vi "P2022 TB INCAR GLOBALES.vi"() -> ()   [LabVIEW 2013]
uses:
  Controles/P2018 Com Control.ctl
  modbusEurotherm P116_485/P2018 Eurotherm Control.ctl
  modbusEurotherm P116_485/4xP116.ctl
  Controles/P2018 Bronkhorst Control.ctl
  serialBronkhorst/_s_TablaBronkhorst.ctl
  Controles/P2018 DisbalTB Control.ctl
  Controles/P2018 Arduino Control.ctl
panel:
  in  "TEMPERATURA":string
  in  "PESO":string
  in  "Cambia_F_f":bool
  out "ERRORES_BONKHORS_f":i32=5 caption="Elapsed Time (s)"
  in  "flowbus_MassFlow":T1={"Dispositivos"=[["3", "NO", "M0000013", "Air", "10", "ln/mn", "0", "0"], ["4", "NO", "M0000014", "Air", "10", "ln/mn", "0", "0"], ["5", "NO", "M0000015", "Air", "10", "ln/mn", "0", "0"], ["6", "NO", "M0000016", "Air", "10", "ln/mn", "0", "0"], ["7", "NO", "M0000017", "Air", "10", "ln/mn", "0", "0"], ["8", "NO", "M0000018", "Air", "10", "ln/mn", "0", "0"]], "NuevosSP"=[["0", "NO", "M0000013", "Air", "1", "ln/mn", "0", "0"], ["0", "NO", "M0000014", "Air", "1", "ln/mn", "0", "0"], ["0", "NO", "M0000015", "Air", "1", "ln/mn", "0", "0"], ["0", "NO", "M0000016", "Air", "1", "ln/mn", "0", "0"], ["0", "NO", "M0000017", "Air", "1", "ln/mn", "0", "0"], ["0", "NO", "M0000018", "Air", "1", "ln/mn", "0", "0"]], "Nodes"=4, "Delay(s)"=0.075}
  in  "ModuloIN":u32=10
  in  "Comments":string
  in  "Cambia_M":bool
  in  "Cambia_D":bool
  in  "Cambia_F_s":bool
  in  "Cambia_T":bool
  in  "Arduino":T3 caption="tarjetaPresion"
  out "Sampling(s)":dbl format="%.1f"
  in  "Disbal":T4 caption="tarjetaPresion"
  out "ERRORES_MOTORES":i32=5 caption="Elapsed Time (s)"
  out "ERRORES_DISBAL":i32=5 caption="Elapsed Time (s)"
  out "ERRORES_BONKHORST_s":i32=5 caption="Elapsed Time (s)"
  out "ERRORES_EUROTHERM":i32=5 caption="Elapsed Time (s)"
  in  "serial_MassFlow":T1={"Dispositivos"=[["3", "NO", "M0000013", "Air", "10", "ln/mn", "0", "0"], ["4", "NO", "M0000014", "Air", "10", "ln/mn", "0", "0"], ["5", "NO", "M0000015", "Air", "10", "ln/mn", "0", "0"], ["6", "NO", "M0000016", "Air", "10", "ln/mn", "0", "0"], ["7", "NO", "M0000017", "Air", "10", "ln/mn", "0", "0"], ["8", "NO", "M0000018", "Air", "10", "ln/mn", "0", "0"]], "NuevosSP"=[["0", "NO", "M0000013", "Air", "1", "ln/mn", "0", "0"], ["0", "NO", "M0000014", "Air", "1", "ln/mn", "0", "0"], ["0", "NO", "M0000015", "Air", "1", "ln/mn", "0", "0"], ["0", "NO", "M0000016", "Air", "1", "ln/mn", "0", "0"], ["0", "NO", "M0000017", "Air", "1", "ln/mn", "0", "0"], ["0", "NO", "M0000018", "Air", "1", "ln/mn", "0", "0"]], "Nodes"=4, "Delay(s)"=0.075}
  in  "P116":T5
  out "Max_t (s)":dbl format="%.1f"
  out "Delta_t (s)":dbl format="%.1f"
  out "Delta_T (C)":dbl format="%.1f"
  in  "TStable?":bool
  out "Comunicaciones":T7={"Flujo_1"="ASRL6::INSTR", "Brk1"=FALSE, "Flujo_2"="ASRL6::INSTR", "Brk2"=FALSE, "Flujo_3"="ASRL6::INSTR", "Brk3"=FALSE, "Flujo_4"="ASRL6::INSTR", "Brk4"=FALSE, "Eurothe"="ASRL6::INSTR", "Eurot"=FALSE, "Balanza"="ASRL6::INSTR", "Bal"=FALSE, "eValPos"="ASRL6::INSTR", "eVal"=FALSE, "flowbus"="ASRL6::INSTR", "fb"=FALSE}
  in  "Saltar":bool
  in  "Pausa":bool
  # "SERIAL"
  # "FLOWBUS"
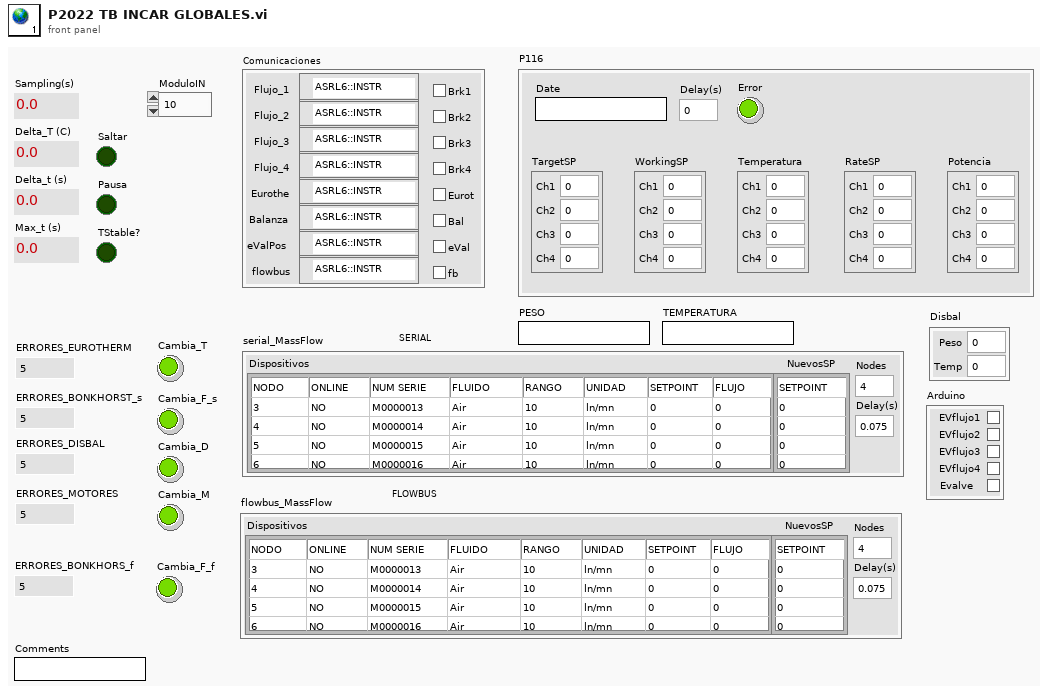
[diagram p1: front panel]
types:
  T1 = typedef "P2018 Bronkhorst Control.ctl" = cluster{"Dispositivos":T2, "NuevosSP":string[][], "Nodes":u32, "Delay(s)":dbl}
  T2 = typedef "_s_TablaBronkhorst.ctl" = string[][]
  T3 = typedef "P2018 Arduino Control.ctl" = cluster{"EVflujo1":bool, "EVflujo2":bool, "EVflujo3":bool, "EVflujo4":bool, "Evalve":bool}
  T4 = typedef "P2018 DisbalTB Control.ctl" = cluster{"Peso":dbl, "Temp":dbl}
  T5 = typedef "P2018 Eurotherm Control.ctl" = cluster{"TargetSP":T6, "WorkingSP":T6, "Temperatura":T6, "Error":bool, "Date":string, "Delay(s)":dbl, "RateSP":T6, "Potencia":T6}
  T6 = typedef "4xP116.ctl" = cluster{"Ch1":dbl, "Ch2":dbl, "Ch3":dbl, "Ch4":dbl}
  T7 = typedef "P2018 Com Control.ctl" = cluster{"Flujo_1":refnum<visa-resource-name>, "Brk1":bool, "Flujo_2":refnum<visa-resource-name>, "Brk2":bool, "Flujo_3":refnum<visa-resource-name>, "Brk3":bool, "Flujo_4":refnum<visa-resource-name>, "Brk4":bool, "Eurothe":refnum<visa-resource-name>, "Eurot":bool, "Balanza":refnum<visa-resource-name>, "Bal":bool, "eValPos":refnum<visa-resource-name>, "eVal":bool, "flowbus":refnum<visa-resource-name>, "fb":bool}
diagram:
